vi "传感器校订.vi"(9 "零点":dbl, 10 "比例":dbl, 11 "传感器":dbl) -> (3 "示值":dbl)   [LabVIEW 2013]
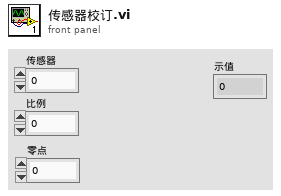
[diagram p1: front panel]
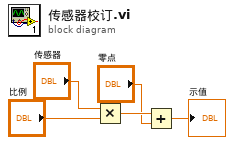
[diagram p0: block diagram]
diagram:
  n1 = Multiply(x="传感器", y="比例") -> (x*y=w5:dbl)
  n2 = Add(x=w5, y="零点") -> (x+y=→"示值":dbl)
